vi "Write Time Stamp.vi"(10 "Start Time":timestamp, 11 "Test Suite Result In":refnum<class "Test Suite Result.lvclass">) -> (3 "Test Suite Result Out":refnum<class "Test Suite Result.lvclass">)   [LabVIEW 2020, in "Test Suite Result.lvclass"]
uses:
  Test Suite Result.lvclass
  Test Suite Result.lvclass/Test Suite Result.ctl
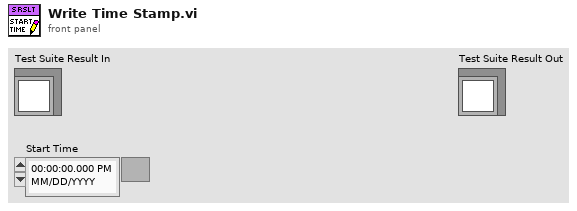
[diagram p1: front panel]
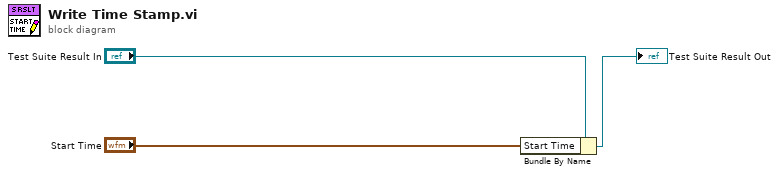
[diagram p0: block diagram]
diagram:
  n1 = Bundle By Name(cluster="Test Suite Result In", "Start Time"="Start Time") -> (→"Test Suite Result Out":refnum<class "Test Suite Result.lvclass">)
